vi "event_common_update_hmi_references.vi"(6 "event_common":refnum<user-event>, 8 "error in (no error)":errorcluster, 11 "hmi_references":T1) -> (0 "error out":errorcluster)   [LabVIEW 2015, in "functional.lvlib"]
uses:
  functional.lvlib
  _controls/event_common.ctl
  _controls/event_common_command.ctl
  public/_controls/hmi_references.ctl
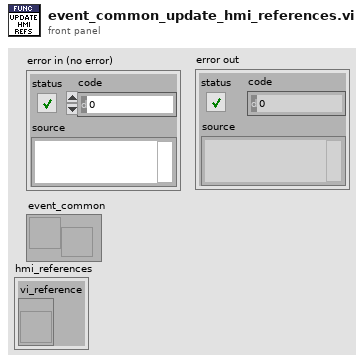
[diagram p1: front panel]
types:
  T1 = typedef "functional.lvlib/hmi_references.ctl" = cluster{"vi_reference":refnum<vi>}
  T2 = typedef "functional.lvlib/event_common_command.ctl" = enum16{"<event_common_cmd>", "update_hmi_references", "die", "<null>"}
  T3 = typedef "functional.lvlib/event_common.ctl" = cluster{"command":T2, "data":variant}
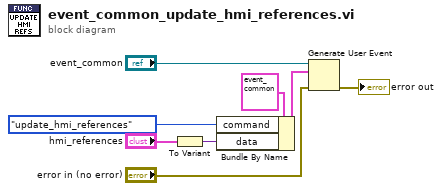
[diagram p0: block diagram]
diagram:
  n1 = To Variant(anything="hmi_references") -> (Variant=w1:variant)
  n2 = Bundle By Name(cluster=T3 {"command"=enum."<event_common_cmd>", "data"=variant} ("event data"), "command"=event_common_command."update_hmi_references", "data"=w1) -> (w4:T3)
  n3 = Generate User Event(user event="event_common", event data cluster=w4, error in="error in (no error)") -> (error out=→"error out":errorcluster)  [unwired: 1 in, 1 out]
